vi "Read Shared Variables - SuNLaMP RTD 6.vi"(9 "channel errors in (no errors)":errorcluster[](array[cluster])) -> (1 "channel errors out":errorcluster[](array[cluster]), 2 "data":dbl[](array[numeric]), 3 "UUIDs":string[](array[string])=["Flow Rate [g/s]", "Density [g/cm^3]", "Return Filter dP [psid]", "Outlet Filter and Flowmeter dp [psid]", "Cooler dP [psid]", "Cooler CO2 In [F]", "Cooler CO2 Out [F]", "Pump Frequency [%]", "Recirc Valve Open [%]"])   [LabVIEW 2017]
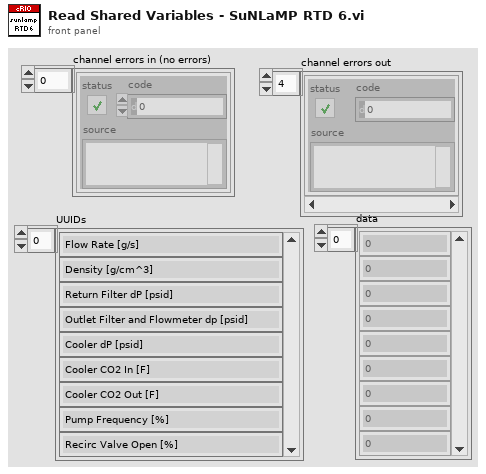
[diagram p1: front panel]
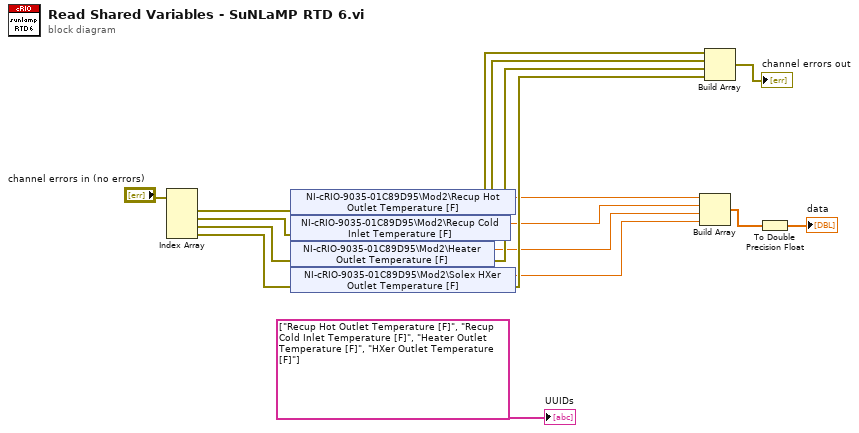
[diagram p0: block diagram]
diagram:
  n1 = Index Array(array="channel errors in (no errors)") -> (element #1=w6:errorcluster, element #2=w5:errorcluster, element #3=w4:errorcluster, element #4=w3:errorcluster)  [unwired: 4 in]
  n2 = shared-variable "NI-cRIO-9035-01C89D95\\Mod2\\Recup Hot Outlet Temperature [F]"(error in=w6) -> (w10:dbl, error out=w14:errorcluster)
  n3 = shared-variable "NI-cRIO-9035-01C89D95\\Mod2\\Recup Cold Inlet Temperature [F]"(error in=w5) -> (w11:dbl, error out=w15:errorcluster)
  n4 = shared-variable "NI-cRIO-9035-01C89D95\\Mod2\\Heater Outlet Temperature [F]"(error in=w4) -> (w12:dbl, error out=w16:errorcluster)
  n5 = shared-variable "NI-cRIO-9035-01C89D95\\Mod2\\Solex HXer Outlet Temperature [F]"(error in=w3) -> (w13:dbl, error out=w17:errorcluster)
  n6 = Build Array(w10, w11, w12, w13) -> (w1:dbl[])
  n7 = Build Array(w14, w15, w16, w17) -> (→"channel errors out":errorcluster[])
  n8 = To Double Precision Float(number=w1) -> (double precision float=→"data":dbl[])
  "UUIDs" <- string[] ["Recup Hot Outlet Temperature [F]", "Recup Cold Inlet Temperature [F]", "Heater Outlet Temperature [F]", "HXer Outlet Temperature [F]"]
